vi "varXNode_Mutate_1_0_0_3.vi"(8 "error in (no error)":errorcluster, 9 "Replies in":string[](array[string]), 10 "Version":T1, 11 "Old State":variant) -> (0 "error out":errorcluster, 1 "Replies out":string[](array[string]), 2 "Version Out":T1, 3 "New State":variant)   [LabVIEW 2017, in "varXNode.xnode"]
uses:
  <vilib>/variable/varXNode.llb/varXNode.xnode
  <vilib>/XNodeSupport/XNodeVersion.ctl
  <vilib>/XNodeSupport/XNodeUShort.ctl
  <vilib>/variable/varXNode.llb/varXNode_old_1_0_0_2.ctl
  <vilib>/variable/varXNode.llb/varXNode_old_1_0_0_3.ctl
  <vilib>/XNodeSupport/NI_XNodeSupport.lvlib
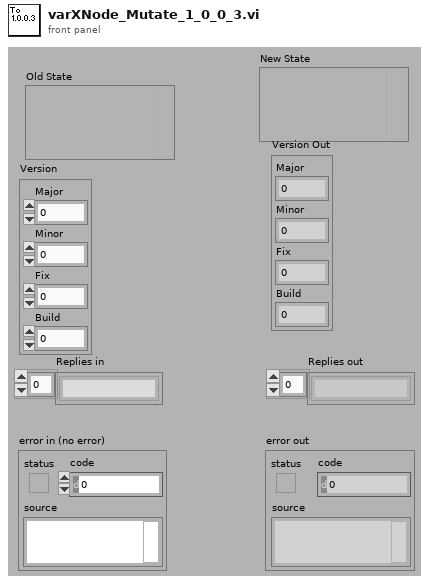
[diagram p1: front panel]
types:
  T1 = typedef "NI_XNodeSupport.lvlib/XNodeVersion.ctl" = cluster{"Major":T2, "Minor":T2, "Fix":T2, "Build":T2}
  T2 = typedef "NI_XNodeSupport.lvlib/XNodeUShort.ctl" = u16
  T3 = typedef "varXNode.xnode/varXNode_old_1_0_0_3.ctl" = cluster{"Write":bool, "ShowTimestamp":bool, "CachedName":string, "CachedTypeDesc":i16[], "CachedFeaturePacks":string[], "Custom Rule":string, "ProjectPath":string, "Bad Code":bool}
  T4 = typedef "varXNode.xnode/varXNode_old_1_0_0_2.ctl" = cluster{"Write":bool, "ShowTimestamp":bool, "CachedName":string, "CachedTypeDesc":i16[], "CachedFeaturePacks":string[], "Custom Rule":string, "ProjectPath":string}
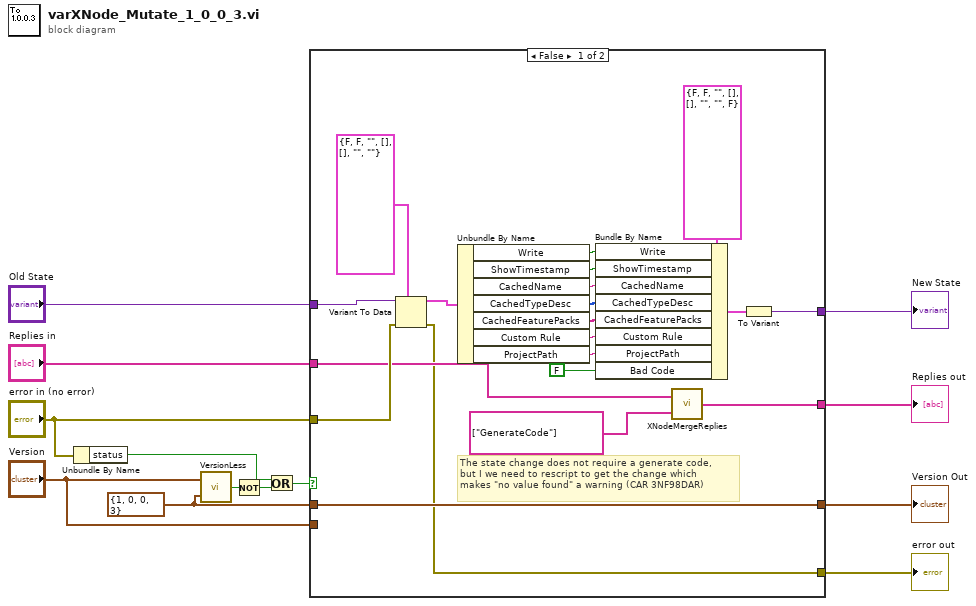
[diagram p0: block diagram]
diagram:
  w12 = T1 {"Major"=1, "Minor"=0, "Fix"=0, "Build"=3} ("y")
  n1 = Unbundle By Name("error in (no error)") -> ("status"=w4:bool)
  n2 = call <vilib>:"VersionLess.vi"("y"=w12, "x"="Version") -> ("x < y?"=w13:bool)
  n3 = Not(x=w13) -> (.not. x?=w3:bool)
  n4 = Or(x=w4, y=w3) -> (x .or. y?=w6:bool)
  n5 = case shown="False" w6 {
    tunnel: w12 -> [w33 _]
    tunnel: [w18 w37] -> w11
    tunnel: "Old State" -> [w32 w37]
    tunnel: [w33 w36] -> w9
    tunnel: "Version" -> [_ w36]
    tunnel: [w14 w35] -> w7
    tunnel: "error in (no error)" -> [w31 w35]
    tunnel: [w15 w34] -> w2
    tunnel: "Replies in" -> [w17 w34]
    frame False {
      # "The state change does not require a generate code,\nbut I we need to rescript to get the change which\nmakes \"no value found\" a warning (CAR 3NF98DAR)"
      n6 = Variant To Data(error in=w31, type=T4 {"Write"=FALSE, "ShowTimestamp"=FALSE, "CachedName"="", "CachedTypeDesc"=[], "CachedFeaturePacks"=[], "Custom Rule"="", "ProjectPath"=""} ("State"), Variant=w32) -> (data=w29:T4, error out=w14:errorcluster)
      n7 = Unbundle By Name(w29) -> ("Write"=w27:bool, "ShowTimestamp"=w26:bool, "CachedName"=w25:string, "CachedTypeDesc"=w24:i16[], "CachedFeaturePacks"=w23:string[], "Custom Rule"=w22:string, "ProjectPath"=w21:string)
      n8 = Bundle By Name(cluster=T3 {"Write"=FALSE, "ShowTimestamp"=FALSE, "CachedName"="", "CachedTypeDesc"=[], "CachedFeaturePacks"=[], "Custom Rule"="", "ProjectPath"="", "Bad Code"=FALSE} ("State"), "Write"=w27, "ShowTimestamp"=w26, "CachedName"=w25, "CachedTypeDesc"=w24, "CachedFeaturePacks"=w23, "Custom Rule"=w22, "ProjectPath"=w21, "Bad Code"=FALSE) -> (w19:T3)
      n9 = call <vilib>:"XNodeMergeReplies.vi"("New Replies"=string[] ["GenerateCode"] ("Replies out"), "Old Replies"=w17) -> ("Merged Replies"=w15:string[])
      n10 = To Variant(anything=w19) -> (Variant=w18:variant)
    }
    frame True {
      # "Either there was an error in,\nor the version is not less than 1.0.0.2.\nPass input values out."
    }
  }
  "New State" <- w11
  "Version Out" <- w9
  "error out" <- w7
  "Replies out" <- w2
